vi "Debug String.vi"(11 "Allow Debugging":bool) -> (3 "Debug String":string)   [LabVIEW 2023, in "VIDoc Printer.lvlib" / "VIDoc Printer.lvclass"]
doc: "Converst the Allow Debug information into a printable String."
uses:
  VIDoc Printer.lvclass
  VIDoc Printer.lvclass/VIDoc Printer.ctl
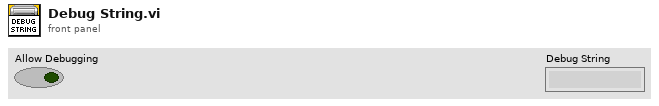
[diagram p1: front panel]
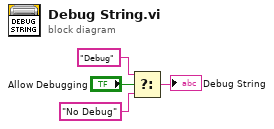
[diagram p0: block diagram]
diagram:
  n1 = Select(t="Debug" ("format string"), s="Allow Debugging", f="No Debug" ("format string")) -> (s? t:f=→"Debug String":string)
